vi "Send Encoder Values to Dashboard.vi"(0 "Distance":string, 1 "Revolutions":string, 2 "Angle":string, 3 "wheel diameteres":dbl, 4 "Encoder Value":dbl) -> ()   [LabVIEW 2013]
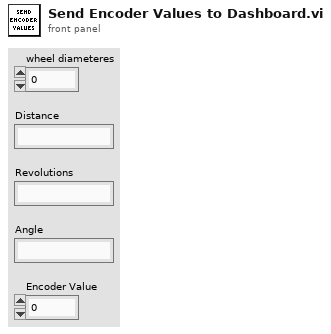
[diagram p1: front panel]
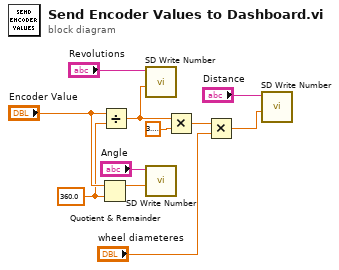
[diagram p0: block diagram]
diagram:
  w1 = 360.0 ("y")
  n1 = Quotient & Remainder(x="Encoder Value", y=w1) -> (x-y*floor(x/y)=w5:dbl)  [unwired: 1 out]
  n2 = Divide(x="Encoder Value", y=w1) -> (x/y=w7:dbl)
  n3 = call <vilib>:"SD Write Number.vi"("Numeric"=w7, "Name"="Revolutions") -> ()  [unwired: 8 in, 2 out]
  n4 = call <vilib>:"SD Write Number.vi"("Numeric"=w5, "Name"="Angle") -> ()  [unwired: 8 in, 2 out]
  n5 = Multiply(x=w7, y=3.141592653589793) -> (x*y=w3:dbl)
  n6 = Multiply(x=w3, y="wheel diameteres") -> (x*y=w9:dbl)
  n7 = call <vilib>:"SD Write Number.vi"("Numeric"=w9, "Name"="Distance") -> ()  [unwired: 8 in, 2 out]
